vi "MiddleLimitSwitch.vi"(10 "Limit Switch":bool, 11 "Motor Command":dbl) -> (3 "Motor Command Out":dbl)   [LabVIEW 2015]
panel:
  out "Enum":enum16{"MoveOffSwitch", "Stop", "Run"}(ring)
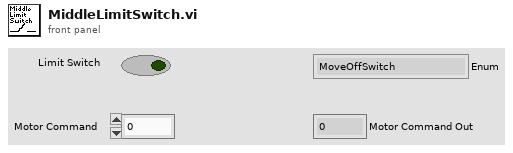
[diagram p1: front panel]
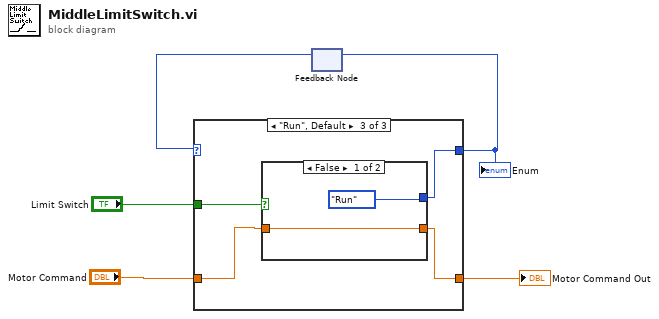
[diagram p0: block diagram]
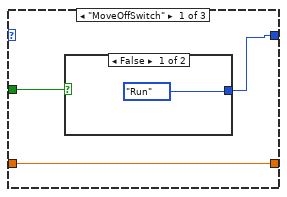
[diagram p2: hidden frame]
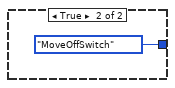
[diagram p3: hidden frame]
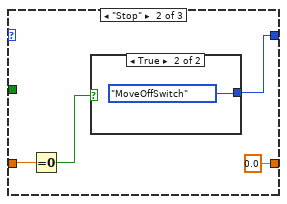
[diagram p4: hidden frame]
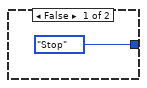
[diagram p5: hidden frame]
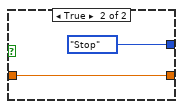
[diagram p6: hidden frame]
diagram:
  n1 = feedback #1() -> (w1:enum16{"MoveOffSwitch", "Stop", "Run"})  [unwired: 1 in]
  n2 = case shown="\"Run\", Default" w1 {
    tunnel: "Motor Command" -> [w8 w14 w18]
    tunnel: [w8 0.0 ("Motor Command") w17] -> w4
    tunnel: [w6 w11 w19] -> w2
    tunnel: "Limit Switch" -> [w7 _ w20]
    frame "MoveOffSwitch" {
      n3 = case shown="False" w7 {
        tunnel: [enum16{"MoveOffSwitch", "Stop", "Run"}."Run" enum16{"MoveOffSwitch", "Stop", "Run"}."MoveOffSwitch"] -> w6
        frame False {
        }
        frame True {
        }
      }
    }
    frame "Stop" {
      n4 = Equal To 0?(x=w14) -> (x = 0?=w13:bool)
      n5 = case shown="True" w13 {
        tunnel: [enum16{"MoveOffSwitch", "Stop", "Run"}."Stop" enum16{"MoveOffSwitch", "Stop", "Run"}."MoveOffSwitch"] -> w11
        frame False {
        }
        frame True {
        }
      }
    }
    frame "Run", Default {
      n6 = case shown="False" w20 {
        tunnel: [enum16{"MoveOffSwitch", "Stop", "Run"}."Run" enum16{"MoveOffSwitch", "Stop", "Run"}."Stop"] -> w19
        tunnel: w18 -> [w21 w23]
        tunnel: [w21 w23] -> w17
        frame False {
        }
        frame True {
        }
      }
    }
  }
  "Motor Command Out" <- w4
  "Enum" <- w2
  n7 = feedback-in #1(w2) -> ()
